vi "Matrix_target.vi"() -> ()   [LabVIEW 2013]
uses:
  <vilib>/Platform/TimedLoop/XDataNode/timing_clust.ctl
  <vilib>/Platform/TimedLoop/XDataNode/nitl_modes.ctl
  <vilib>/Platform/TimedLoop/XDataNode/wakeup.ctl
  <vilib>/rvi/Emulation/niFpgaSctlEmulationGetInTimedLoop.vi
  <vilib>/rvi/Emulation/niFpgaEmulationReportErrorSimple.vi
  <vilib>/rvi/Emulation/niFpgaGetClockAttributes.vi
  <vilib>/rvi/Emulation/niFpgaCriticalErrorInLSC.vi
  <vilib>/rvi/eio/common/nirviEmuTemplateMethod_errors.vi
  <vilib>/rvi/Emulation/niFpgaProcessEmulError.vi
  <vilib>/Platform/TimedLoop/XDataNode/XDataNode.xnode
  <vilib>/eio/EIONode/EIONode.xnode
  <vilib>/Platform/TimedLoop/XDataNode/XDNodeRunTimeDep.lvlib
panel:
  in  "1_EXTCLK_divider":i16
  in  "IO Module\\Local_Supply_Select":u8
  in  "54":i16=53
  in  "36":i16=35
  in  "18":i16=17
  in  "72":i16=53
  in  "71":i16=53
  in  "17":i16=17
  in  "35":i16=35
  in  "53":i16=53
  in  "0_WE divider":i32=10
  in  "10_Rise/Fall divider":i32=3
  in  "75_Stop":i16=57
  out "Data_Array":bool[](array[boolean])
  in  "Send_Request":bool
  in  "DataLow":u64
  out "ACK":bool[](array[boolean])
  in  "/Reset_Bar":bool
  out "Sclk":bool
  in  "DataUp":u64
  in  "100_Sclk_divider":i32=25
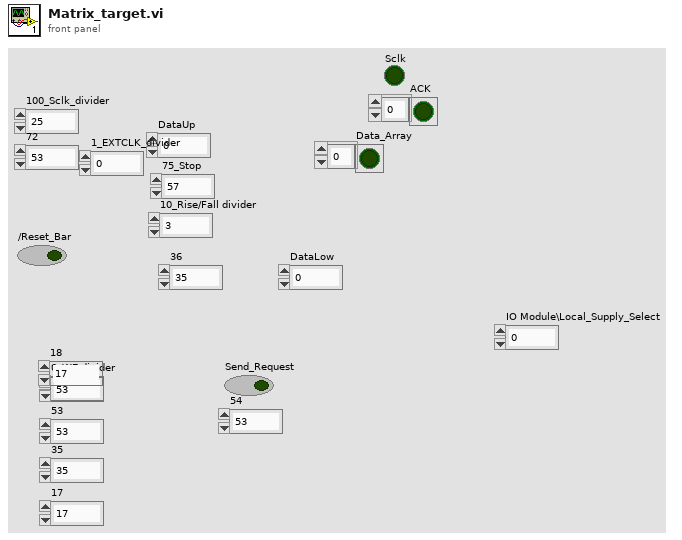
[diagram p1: front panel]
types:
  T1 = typedef "XDNodeRunTimeDep.lvlib/timing_clust.ctl" = cluster{"Expected End [f-1]":u64, "Actual End [f-1]":u64, "Finished Late? [f-1]":bool, "Expected End [i-1]":u64, "Actual End [i-1]":u64, "Finished Late? [i-1]":bool, "Expected Start [i]":u64, "Actual Start [i]":u64, "Expected Start [f]":u64, "Actual Start [f]":u64, "Source Name":string, "Structure Name":string, "Period":i64, "Deadline":i64, "Offset":i64, "Start":i64, "Priority":i32, "Timeout":i32, "Mode":T2, "Wakeup Reason":T3, "Error":errorcluster, "Source Type":string, "Secondary Source Type":string, "Global End Time":u64, "Global Start Time":u64, "Frame Duration":u64, "Iteration Duration":u64, "Assigned CPU":i32, "I/O Scan Engine Mode":u32}
  T2 = typedef "XDNodeRunTimeDep.lvlib/nitl_modes.ctl" = enum32{"No Change", "Process missed periods, maintain original phase", "Discard missed periods, maintain original phase", "Process missed periods, ignore original phase", "Discard missed periods, ignore original phase"}
  T3 = typedef "XDNodeRunTimeDep.lvlib/wakeup.ctl" = enum32{"Normal", "Aborted", "Asynchronous wakeup", "Timing source error", "Timed loop error", "Timeout"}
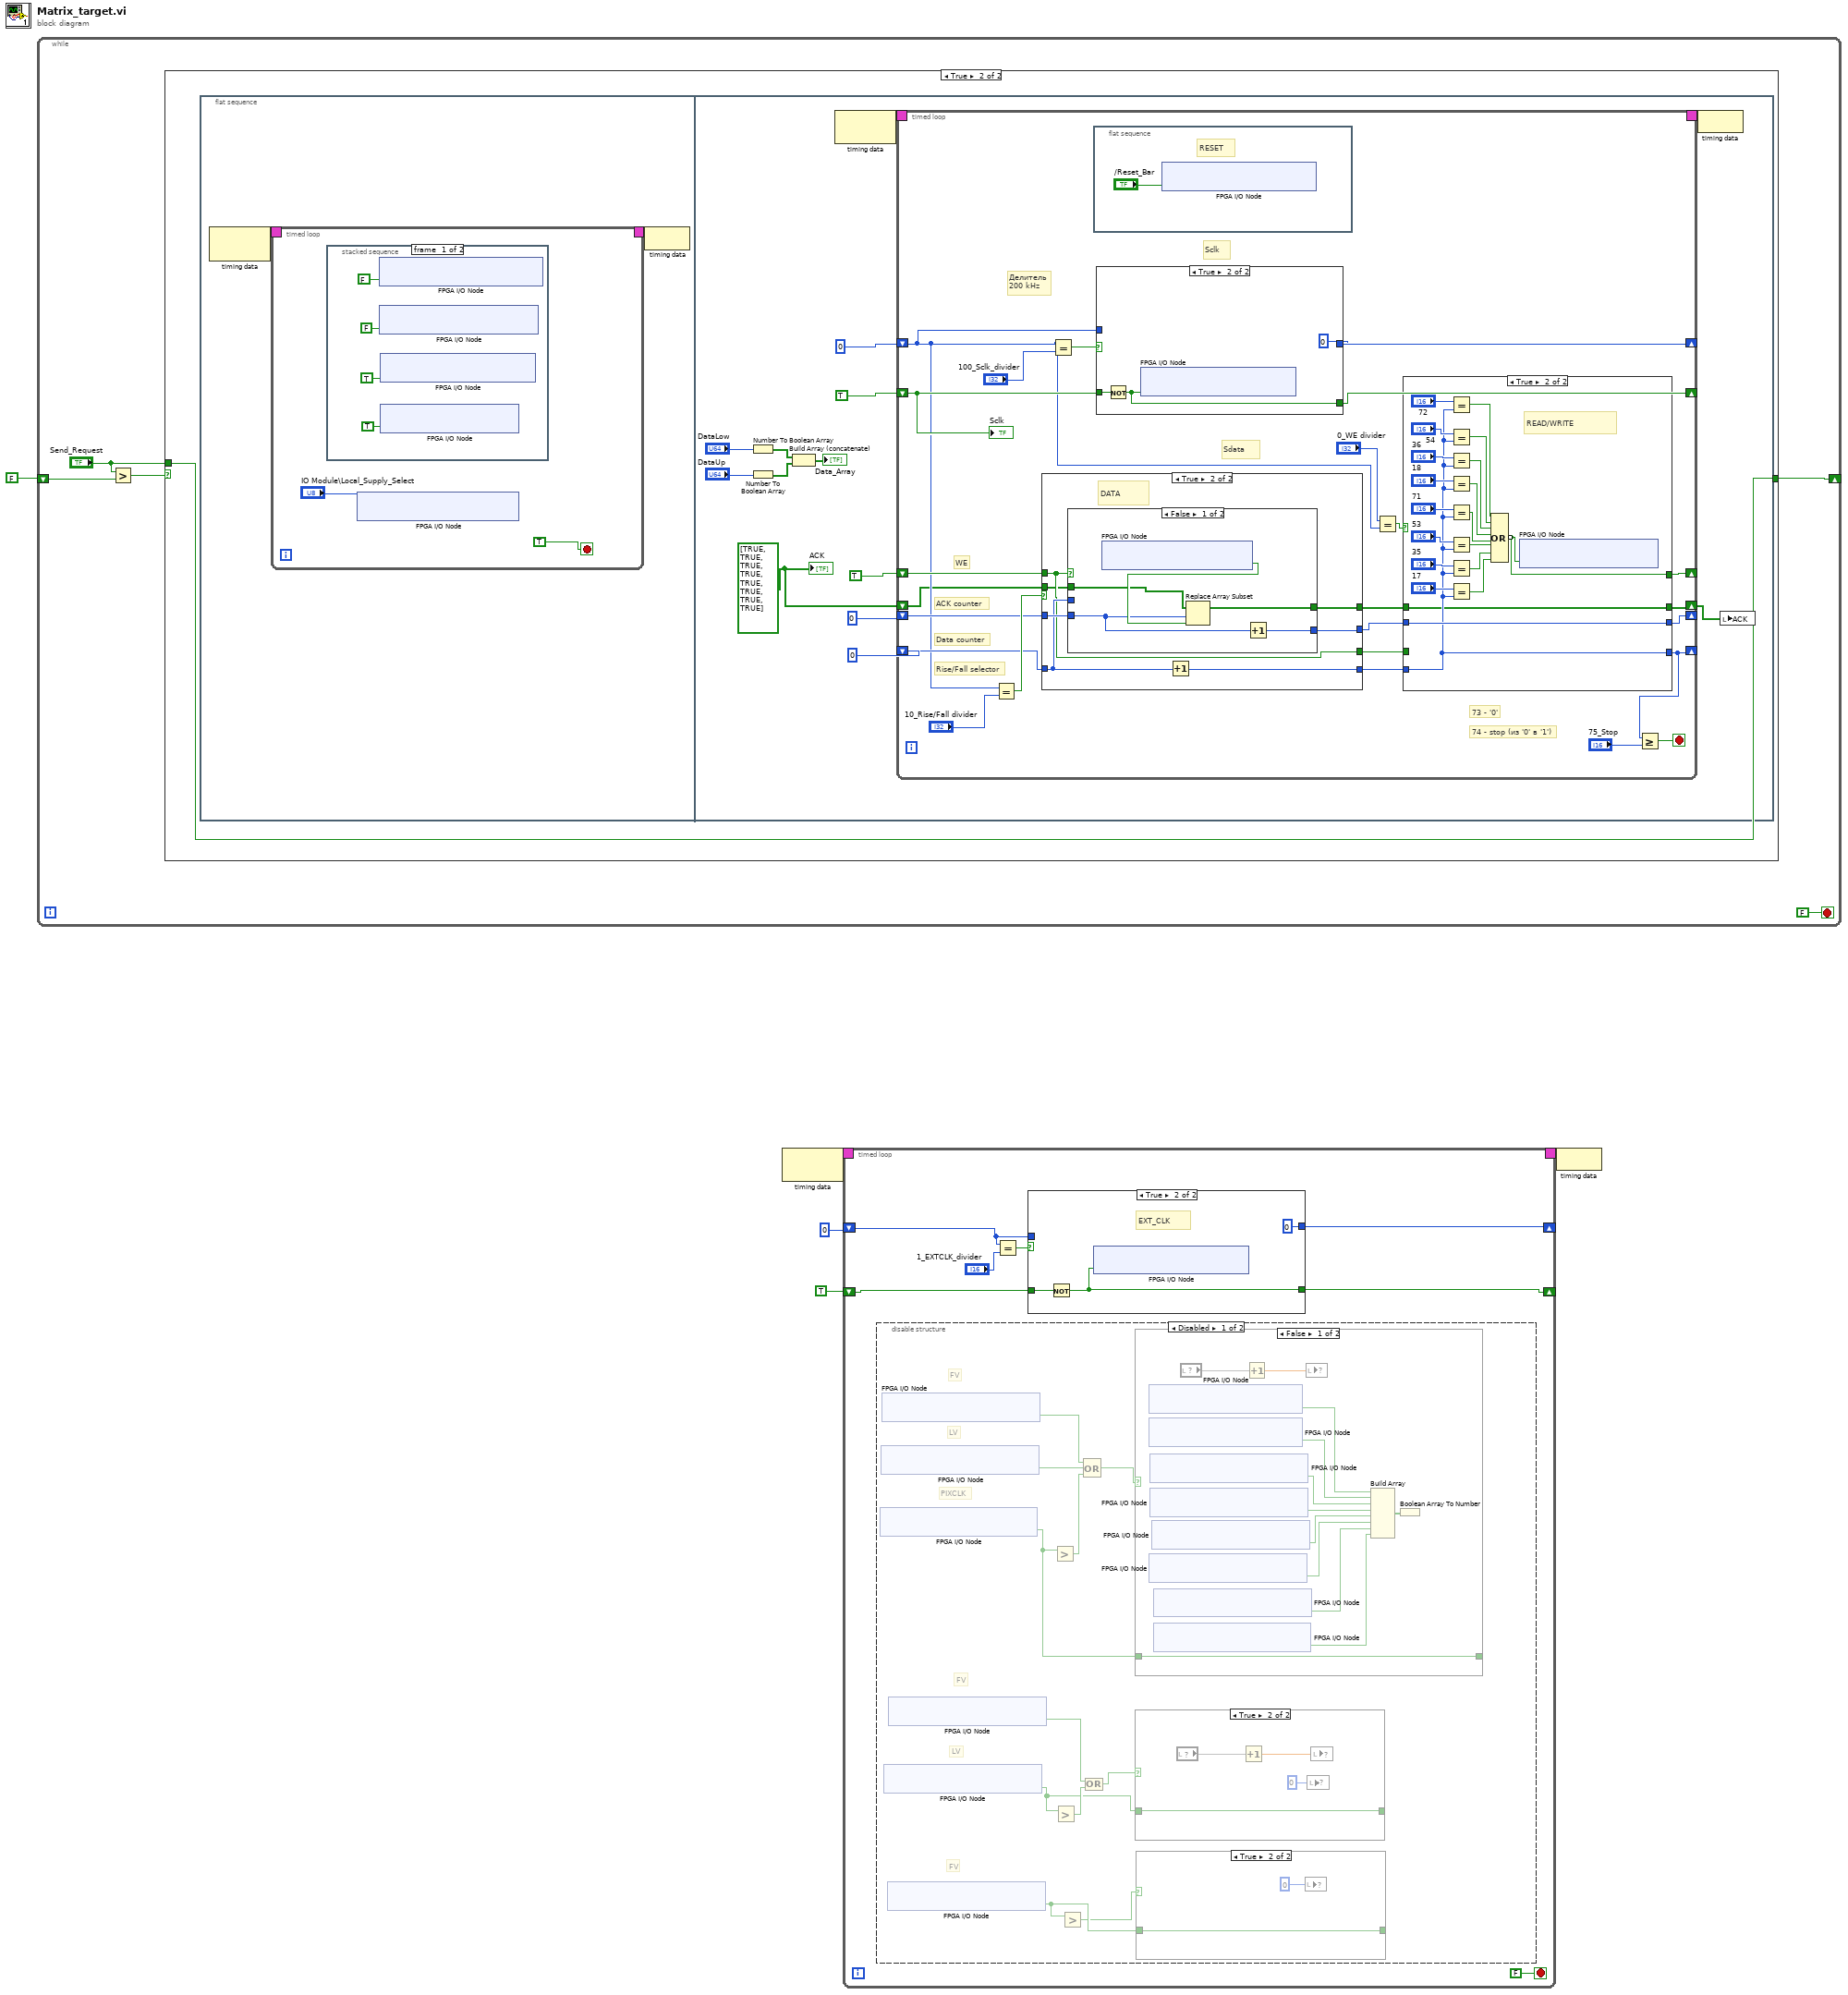
[diagram p0: block diagram]
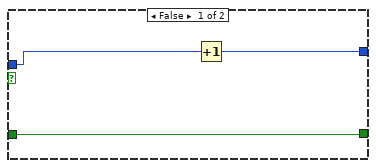
[diagram p2: hidden frame]
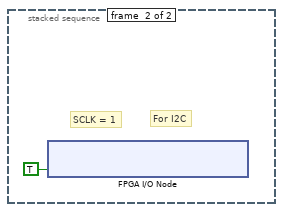
[diagram p8: hidden frame]
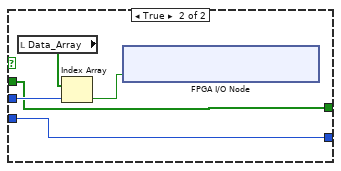
[diagram p11: hidden frame]
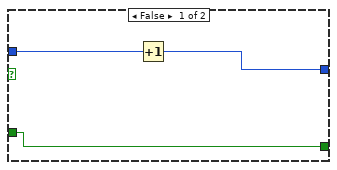
[diagram p12: hidden frame]
diagram:
  n1 = while {
    shift-right: [w9] -> _
    shift-left: FALSE ("Send_Request") -> [w8]
    stop <- FALSE stop-if-true
    n2 = Greater?(x="Send_Request", y=w8) -> (0:w7:bool)
    n3 = case shown="True" w7 {
      tunnel: "Send_Request" -> [w11 w12]
      tunnel: [w11 w12] -> w9
      frame False {
      }
      frame True {
        n4 = flat-sequence {
          frame #0 {
            n5 = node-c288() -> (w14:T1)  [unwired: 1 in]
            n6 = timed-loop {
              timing: w14 -> [_]
              timing-out: [_] -> w13
              stop <- TRUE stop-if-true
              n7 = stacked-sequence {
                frame #0 {
                  n8 = xnode "FPGA I/O Node"("IO Module\\DDCA_DIO16-23_WE"=FALSE ("IO Module\\DDCA_DIO16-23_WE")) -> ()  [unwired: 1 in, 1 out]
                  n9 = xnode "FPGA I/O Node"("IO Module\\DDCA_DIO8-15_WE"=FALSE ("IO Module\\DDCA_DIO8-15_WE")) -> ()  [unwired: 1 in, 1 out]
                  n10 = xnode "FPGA I/O Node"("IO Module\\DDCA_DIO0-7_WE"=TRUE ("IO Module\\DDCA_DIO0-7_WE")) -> ()  [unwired: 1 in, 1 out]
                  n11 = xnode "FPGA I/O Node"("IO Module\\DDCA_PFI_WE"=TRUE ("IO Module\\DDCA_DIO0-7_WE")) -> ()  [unwired: 1 in, 1 out]
                }
                frame #1 {
                  # "For I2C"
                  # "SCLK = 1"
                  n12 = xnode "FPGA I/O Node"("IO Module\\DDCA_DIO6_Write"=TRUE ("IO Module\\DDCA_DIO6_Write")) -> ()  [unwired: 1 in, 1 out]
                }
              }
              n13 = xnode "FPGA I/O Node"("IO Module\\Local_Supply_Select"="IO Module\\Local_Supply_Select") -> ()  [unwired: 1 in, 1 out]
            }
            n14 = node-c288(w13) -> ()
          }
          frame #1 {
            w26 = bool[] [TRUE, TRUE, TRUE, TRUE, TRUE, TRUE, TRUE, TRUE] ("ACK")
            n15 = Number To Boolean Array(number="DataLow") -> (Boolean array=w33:bool[])
            n16 = Number To Boolean Array(number="DataUp") -> (Boolean array=w32:bool[])
            n17 = Build Array (concatenate)(w33, w32) -> (→"Data_Array":bool[])
            n18 = node-c288() -> (w39:T1)  [unwired: 1 in]
            n19 = timed-loop {
              timing: w39 -> [_]
              timing-out: [_] -> w38
              shift-right: [w62] -> _
              shift-left: 0 -> [w51]
              shift-right: [w61] -> _
              shift-left: TRUE ("IO Module\\DDCA_DIO0_Write") -> [w58]
              shift-right: [w48] -> _
              shift-left: i16 0 -> [w56]
              shift-right: [w46] -> _
              shift-left: i16 0 -> [w55]
              shift-right: [w45] -> _
              shift-left: TRUE -> [w54]
              shift-right: [w41] -> w27
              shift-left: w26 -> [w40]
              stop <- w43 stop-if-true
              # "Rise/Fall selector"
              # "WE"
              # "Data counter"
              # "ACK counter"
              # "74 - stop (из '0' в '1')"
              # "73 - '0'"
              # "Sdata"
              # "Sclk"
              # "Делитель\n200 kHz"
              n20 = Equal?(x=w51, y="10_Rise/Fall divider") -> (x = y?=w57:bool)
              n21 = case shown="True" w57 {
                tunnel: [w90 w94] -> w49
                tunnel: w56 -> [w90 w96]
                tunnel: w55 -> [w91 w98]
                tunnel: [w91 w97] -> w47
                tunnel: w54 -> [w89 w95]
                tunnel: [w89 w95] -> w44
                tunnel: [w88 w93] -> w42
                tunnel: w40 -> [w88 w92]
                frame False {
                }
                frame True {
                  # "DATA"
                  n22 = case shown="False" w95 {
                    tunnel: w98 -> [w102 w108]
                    tunnel: [w101 w108] -> w97
                    tunnel: w96 -> [_ w107]
                    tunnel: [w100 w104] -> w93
                    tunnel: w92 -> [w99 w104]
                    frame False {
                      n23 = xnode "FPGA I/O Node"() -> ("IO Module\\DDCA_PFI1_Read"=w103:bool)  [unwired: 1 in, 1 out]
                      n24 = Replace Array Subset(array=w99, new element=w103, index=w102) -> (w100:bool[])
                      n25 = Increment(x=w102) -> (x+1=w101:i16)
                    }
                    frame True {
                      n26 = local read "Data_Array"() -> (w106:bool[])
                      n27 = Index Array(array=w106, index=w107) -> (element=w105:bool)
                      n28 = xnode "FPGA I/O Node"("IO Module\\DDCA_PFI1_Write"=w105) -> ()  [unwired: 1 in, 1 out]
                    }
                  }
                  n29 = Increment(x=w96) -> (x+1=w94:i16)
                }
              }
              n30 = Equal?(x=w51, y="100_Sclk_divider") -> (x = y?=w63:bool)
              n31 = flat-sequence {
                frame #0 {
                  # "RESET"
                  n32 = xnode "FPGA I/O Node"("IO Module\\DDCA_DIO5_Write"="/Reset_Bar") -> ()  [unwired: 1 in, 1 out]
                }
              }
              n33 = case shown="True" w63 {
                tunnel: [w111 0] -> w62
                tunnel: w51 -> [w112 _]
                tunnel: w58 -> [w110 w114]
                tunnel: [w110 w113] -> w61
                frame False {
                  n34 = Increment(x=w112) -> (x+1=w111:i32)
                }
                frame True {
                  n35 = Not(x=w114) -> (.not. x?=w113:bool)
                  n36 = xnode "FPGA I/O Node"("IO Module\\DDCA_DIO6_Write"=w113) -> ()  [unwired: 1 in, 1 out]
                }
              }
              n37 = Equal?(x="0_WE divider", y=w51) -> (x = y?=w50:bool)
              n38 = case shown="True" w50 {
                tunnel: w49 -> [w66 w73]
                tunnel: [w66 w73] -> w48
                tunnel: [w67 w79] -> w46
                tunnel: w47 -> [w67 w79]
                tunnel: [w65 w78] -> w45
                tunnel: w44 -> [w65 _]
                tunnel: w42 -> [w64 w68]
                tunnel: [w64 w68] -> w41
                frame False {
                }
                frame True {
                  # "READ/WRITE"
                  n39 = Equal?(x="72", y=w73) -> (x = y?=w72:bool)
                  n40 = Equal?(x="54", y=w73) -> (x = y?=w69:bool)
                  n41 = Equal?(x="36", y=w73) -> (x = y?=w71:bool)
                  n42 = Equal?(x="18", y=w73) -> (x = y?=w70:bool)
                  n43 = Equal?(x="71", y=w73) -> (x = y?=w80:bool)
                  n44 = Equal?(x="53", y=w73) -> (x = y?=w83:bool)
                  n45 = Equal?(x="35", y=w73) -> (x = y?=w85:bool)
                  n46 = Equal?(x="17", y=w73) -> (x = y?=w87:bool)
                  n47 = Compound Arithmetic op=OR(w72, w69, w71, w70, w80, w83, w85, w87) -> (invert w78:bool)
                  n48 = xnode "FPGA I/O Node"("IO Module\\DDCA_PFI_WE"=w78) -> ()  [unwired: 1 in, 1 out]
                }
              }
              n49 = Greater Or Equal?(x=w48, y="75_Stop") -> (x >= y?=w43:bool)
              "Sclk" <- w58
            }
            n50 = node-c288(w38) -> ()
            n51 = local write "ACK"(w27) -> ()
            "ACK" <- w26
          }
        }
      }
    }
  }
  n52 = node-c288() -> (w4:T1)  [unwired: 1 in]
  n53 = timed-loop {
    timing: w4 -> [_]
    timing-out: [_] -> w3
    shift-right: [w124] -> _
    shift-left: TRUE -> [w125]
    shift-right: [w121] -> _
    shift-left: i16 0 -> [w122]
    stop <- FALSE stop-if-true
    n54 = disable-structure shown="Disabled" {
      frame Disabled {
        # "FV"
        # "LV"
        # "FV"
        # "PIXCLK"
        # "LV"
        # "FV"
        n55 = xnode "FPGA I/O Node"() -> ("IO Module\\DDCA_DIO17_Read"=w137:bool)  [unwired: 1 in, 1 out]
        n56 = xnode "FPGA I/O Node"() -> ("IO Module\\DDCA_DIO22_Read"=w142:bool)  [unwired: 1 in, 1 out]
        n57 = xnode "FPGA I/O Node"() -> ("IO Module\\DDCA_DIO23_Read"=w141:bool)  [unwired: 1 in, 1 out]
        n58 = xnode "FPGA I/O Node"() -> ("IO Module\\DDCA_DIO22_Read"=w135:bool)  [unwired: 1 in, 1 out]
        n59 = xnode "FPGA I/O Node"() -> ("IO Module\\DDCA_DIO23_Read"=w134:bool)  [unwired: 1 in, 1 out]
        n60 = xnode "FPGA I/O Node"() -> ("IO Module\\DDCA_DIO23_Read"=w139:bool)  [unwired: 1 in, 1 out]
        n61 = Greater?(x=w137) -> (0:w143:bool)  [unwired: 1 in]
        n62 = Greater?(x=w135) -> (0:w136:bool)  [unwired: 1 in]
        n63 = Greater?(x=w134) -> (0:w133:bool)  [unwired: 1 in]
        n64 = Compound Arithmetic op=OR(w141, w142, w143) -> (w140:bool)
        n65 = Compound Arithmetic op=OR(w139, w136) -> (w138:bool)
        n66 = case shown="False" w140 {
          tunnel: [w163 w164] -> _
          tunnel: w137 -> [w163 w164]
          frame False {
            n67 = xnode "FPGA I/O Node"() -> ("IO Module\\DDCA_DIO8_Read"=w160:bool)  [unwired: 1 in, 1 out]
            n68 = xnode "FPGA I/O Node"() -> ("IO Module\\DDCA_DIO9_Read"=w159:bool)  [unwired: 1 in, 1 out]
            n69 = xnode "FPGA I/O Node"() -> ("IO Module\\DDCA_DIO13_Read"=w155:bool)  [unwired: 1 in, 1 out]
            n70 = xnode "FPGA I/O Node"() -> ("IO Module\\DDCA_DIO10_Read"=w158:bool)  [unwired: 1 in, 1 out]
            n71 = xnode "FPGA I/O Node"() -> ("IO Module\\DDCA_DIO11_Read"=w157:bool)  [unwired: 1 in, 1 out]
            n72 = xnode "FPGA I/O Node"() -> ("IO Module\\DDCA_DIO12_Read"=w156:bool)  [unwired: 1 in, 1 out]
            n73 = xnode "FPGA I/O Node"() -> ("IO Module\\DDCA_DIO13_Read"=w153:bool)  [unwired: 1 in, 1 out]
            n74 = xnode "FPGA I/O Node"() -> ("IO Module\\DDCA_DIO13_Read"=w154:bool)  [unwired: 1 in, 1 out]
            n75 = local read item#-1() -> (w162)
            n76 = Increment(x=w162) -> (x+1=w161:dbl)
            n77 = local write item#-1(w161) -> ()
            n78 = Build Array(w160, w159, w158, w157, w156, w155, w154, w153) -> (w152:bool[])
            n79 = Boolean Array To Number(Boolean array=w152) -> ()  [unwired: 1 out]
          }
          frame True {
          }
        }
        n80 = case shown="True" w138 {
          tunnel: w135 -> [w147 w151]
          tunnel: [w147 w151] -> _
          frame False {
          }
          frame True {
            n81 = local read item#-1() -> (w150)
            n82 = Increment(x=w150) -> (x+1=w149:dbl)
            n83 = local write item#-1(i16 0 ("Pix")) -> ()
            n84 = local write item#-1(w149) -> ()
          }
        }
        n85 = case shown="True" w133 {
          tunnel: w134 -> [w144 w146]
          tunnel: [w144 w146] -> _
          frame False {
          }
          frame True {
            n86 = local write item#-1(i16 0 ("Lines")) -> ()
          }
        }
      }
      frame Enabled {
      }
    }
    n87 = Equal?(x=w122, y="1_EXTCLK_divider") -> (x = y?=w123:bool)
    n88 = case shown="True" w123 {
      tunnel: w125 -> [w127 w132]
      tunnel: [w127 w131] -> w124
      tunnel: w122 -> [w129 _]
      tunnel: [w128 i16 0] -> w121
      frame False {
        n89 = Increment(x=w129) -> (x+1=w128:i16)
      }
      frame True {
        # "EXT_CLK"
        n90 = Not(x=w132) -> (.not. x?=w131:bool)
        n91 = xnode "FPGA I/O Node"("IO Module\\DDCA_DIO7_Write"=w131) -> ()  [unwired: 1 in, 1 out]
      }
    }
  }
  n92 = node-c288(w3) -> ()
